vi "DAQmx Create Channel (CI-Velocity-Angular).vi"(0 "task in":refnum<k21>, 1 "maximum value":dbl=1.0, 2 "minimum value":dbl, 5 "counter":tag, 6 "decoding type":i32(ring)=10092 items=["X1"=10090, "X2"=10091, "X4"=10092, "Two Pulse Counting"=10313], 7 "name to assign":string, 9 "units":i32(ring)=16080 items=["RPM"=16080, "Radians/s"=16081, "Degrees/s"=16082, "From Custom Scale"=10065], 11 "error in":errorcluster, 12 "custom scale name":tag, 13 "pulses per revolution":u32=24) -> (4 "task out":refnum<k21>, 15 "error out":errorcluster)   [LabVIEW 2013]
doc: "Creates a channel to measure the angular velocity of a digital signal. With the exception of devices that support multi-counter tasks, you can create only one counter input channel at a time with this VI because a task can contain only one counter input channel. To read from multiple counters simultaneously, use a separate task for each counter. Connect the input signal to the default input terminal of the counter unless you select a different input terminal."
uses:
  <resource>/objmgr/daqmx.rc
panel:
  # "input limits"
  # "encoder info"
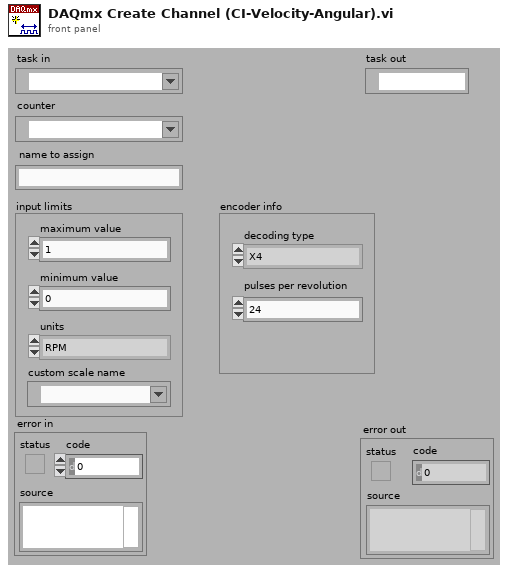
[diagram p1: front panel]
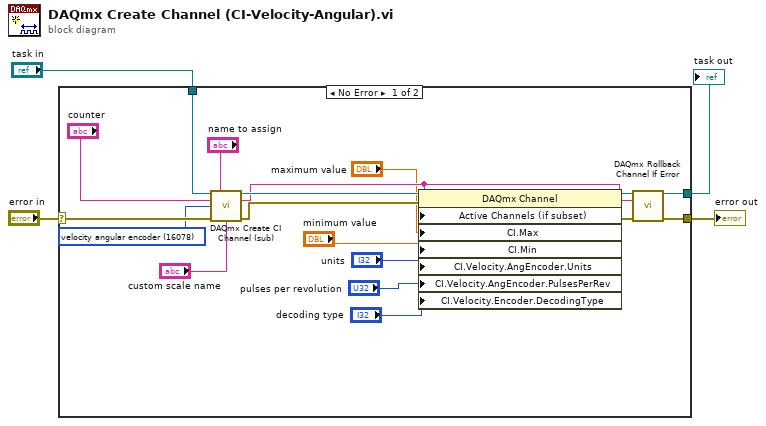
[diagram p0: block diagram]
diagram:
  n1 = case shown="No Error" "error in" {
    selector: "error in" -> [w21 w23]
    tunnel: "task in" -> [w22 w24]
    tunnel: [w15 w24] -> w2
    tunnel: [w14 w23] -> w1
    frame No Error {
      w12 = 16078 items=["count events"=10125, "frequency"=10179, "period"=10256, "pulse width"=10359, "semi period"=10289, "two edge separation"=10267, "angular encoder"=10360, "linear encoder"=10361, "velocity angular encoder"=16078, "velocity linear encoder"=16079] ("measurement type")
      n2 = call "DAQmx Create CI Channel (sub).vi"("task in"=w22, "virtual channel name"="name to assign", "physical channel name"="counter", "measurement type"=w12, "error in"=w21, "custom scale"="custom scale name") -> ("task out"=w17:refnum<k21>, "channel names"=w8:string, "error out"=w19:errorcluster)  [unwired: 7 out]
      n3 = property class="DAQmx Channel"(reference=w17, error in=w19, "Active Channels (if subset)"=w8, "CI.Max"="maximum value", "CI.Min"="minimum value", "CI.Velocity.AngEncoder.Units"="units", "CI.Velocity.AngEncoder.PulsesPerRev"="pulses per revolution", "CI.Velocity.Encoder.DecodingType"="decoding type") -> (reference out=w16:refnum<k21>, error out=w13:errorcluster)
      n4 = call "DAQmx Rollback Channel If Error.vi"("task in"=w16, "channel names"=w8, "error in"=w13) -> ("task out"=w15:refnum<k21>, "error out"=w14:errorcluster)  [unwired: 11 out]
    }
    frame Error {
    }
  }
  "error out" <- w1
  "task out" <- w2
